vi "pulsePIP.vi"(8 "error in (no error)":errorcluster) -> (0 "error out":errorcluster, 3 "PULSE-17":string)   [LabVIEW 2018]
uses:
  Global_1259.vi
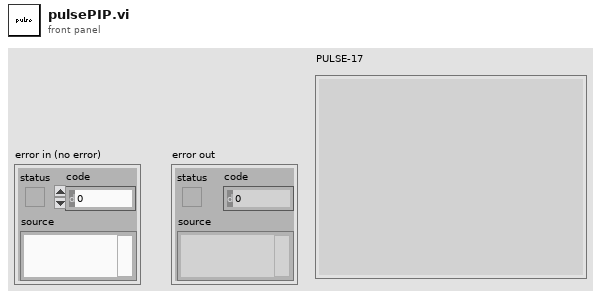
[diagram p1: front panel]
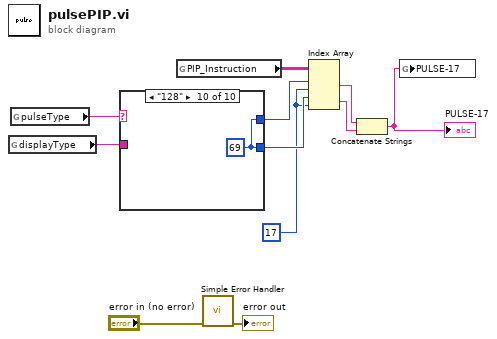
[diagram p0: block diagram]
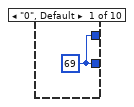
[diagram p2: hidden frame]
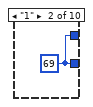
[diagram p3: hidden frame]
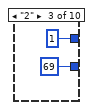
[diagram p4: hidden frame]
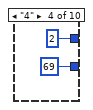
[diagram p5: hidden frame]
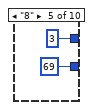
[diagram p6: hidden frame]
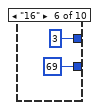
[diagram p7: hidden frame]
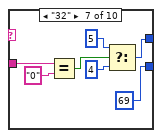
[diagram p8: hidden frame]
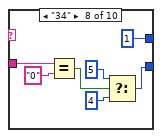
[diagram p9: hidden frame]
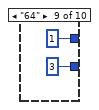
[diagram p10: hidden frame]
diagram:
  w4 = 17
  n1 = global read "Global_1259.vi" "displayType"() -> (w9:string)
  n2 = global read "Global_1259.vi" "pulseType"() -> (w8:string)
  n3 = case shown="\"128\"" w8 {
    tunnel: [w12 w13 69 69 69 69 69 w32 3 w38] -> w7
    tunnel: [w12 w13 1 2 3 3 w22 1 1 w38] -> w6
    tunnel: w9 -> [_ _ _ _ _ _ w24 w29 _ _]
    frame "0", Default {
      w12 = 69
    }
    frame "1" {
      w13 = 69
    }
    frame "2" {
    }
    frame "4" {
    }
    frame "8" {
    }
    frame "16" {
    }
    frame "32" {
      n4 = Equal?(x=w24, y="0") -> (x = y?=w28:bool)
      n5 = Select(t=5, s=w28, f=4) -> (s? t:f=w22:i32)
    }
    frame "34" {
      n6 = Equal?(x=w29, y="0") -> (x = y?=w35:bool)
      n7 = Select(t=5, s=w35, f=4) -> (s? t:f=w32:i32)
    }
    frame "64" {
    }
    frame "128" {
      w38 = 69
    }
  }
  n8 = global read "Global_1259.vi" "PIP_Instruction"() -> (w2:string[][])
  n9 = call <vilib>:"Simple Error Handler.vi"("error in (no error)"="error in (no error)") -> ("error out"=→"error out":errorcluster)  [unwired: 4 in, 4 out]
  n10 = Index Array(array=w2, index (row) #1=w6, index (col) #1=w4, index (row) #2=w7, index (col) #2=w4) -> (element #1=w5:string, element #2=w1:string)
  n11 = Concatenate Strings(w5, w1) -> (w3:string)
  "PULSE-17" <- w3
  n12 = global write "Global_1259.vi" "PULSE-17"(w3) -> ()
